vi "Write Command.vi"(8 "error in":errorcluster, 10 "command":string, 11 "GOLPI ref. in":T1={"pipe handle"={"lv_proc.dll file path"=path "", "process instance handle"=[], "debug mode"=FALSE, "debug data"=[]}, "fast read timeout [ms]"=500, "fast read settle time [ms]"=10, "fast read to multiple [ms]"=1, "max elements per input line"=100, "slow read timeout [ms]"=5000, "stdin double format specifier"="", "max elements per stdout output column"=100, "console mode bitstream"=FALSE, "bitstream first read timeout [ms]"=1000, "bitstream read timeout [ms]"=50, "struct transfer possible"=FALSE, "matlab mode"=FALSE}) -> (0 "error out":errorcluster, 3 "GOLPI ref. out":T1={"pipe handle"={"lv_proc.dll file path"=path "", "process instance handle"=[], "debug mode"=FALSE, "debug data"=[]}, "fast read timeout [ms]"=500, "fast read settle time [ms]"=10, "fast read to multiple [ms]"=1, "max elements per input line"=100, "slow read timeout [ms]"=5000, "stdin double format specifier"="", "max elements per stdout output column"=100, "console mode bitstream"=FALSE, "bitstream first read timeout [ms]"=1000, "bitstream read timeout [ms]"=50, "struct transfer possible"=FALSE, "matlab mode"=FALSE})   [LabVIEW 2020, in "GOLPI library.lvlib"]
doc: "Sends command to GNU Octave. End of line is added automatically if missing.\n\n---\nGOLPI works only with lv_proc.dll library, which is part of vipm package or should be delivered together with packed library. Placement of this dll is selected in terminal of Start GNU Octave.vi."
uses:
  GOLPI library.lvlib
  GOLPI reference Type Def.ctl
  Pipe Handle.ctl
  LV Process library.lvlib
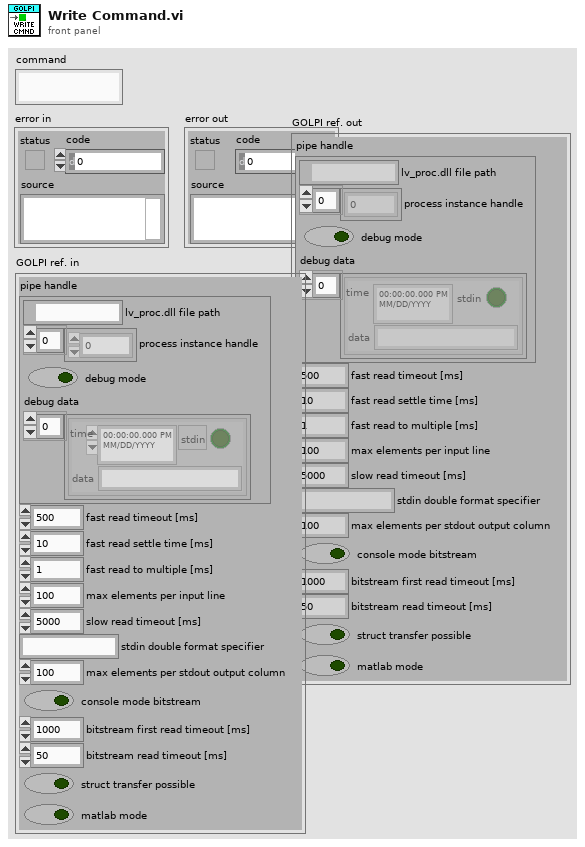
[diagram p1: front panel]
types:
  T1 = typedef "GOLPI library.lvlib/GOLPI reference Type Def.ctl" = cluster{"pipe handle":T2, "fast read timeout [ms]":u32, "fast read settle time [ms]":u32, "fast read to multiple [ms]":u32, "max elements per input line":u32, "slow read timeout [ms]":u32, "stdin double format specifier":string, "max elements per stdout output column":u32, "console mode bitstream":bool, "bitstream first read timeout [ms]":u32, "bitstream read timeout [ms]":u32, "struct transfer possible":bool, "matlab mode":bool}
  T2 = typedef "LV Process library.lvlib/Pipe Handle.ctl" = cluster{"lv_proc.dll file path":path, "process instance handle":u32[], "debug mode":bool, "debug data":cluster{"time":timestamp, "stdin":bool, "data":string}[]}
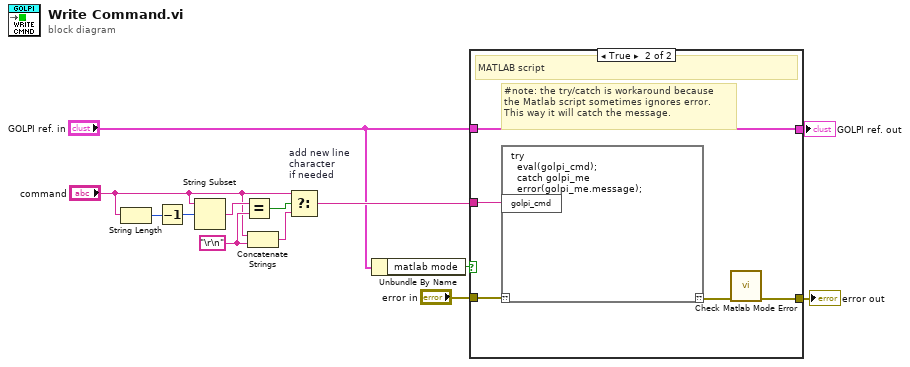
[diagram p0: block diagram]
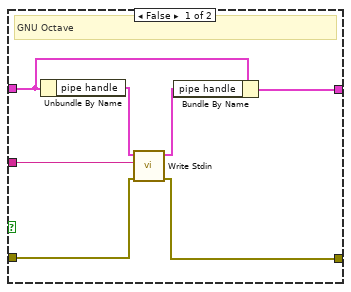
[diagram p2: hidden frame]
diagram:
  w8 = "\r\n"
  n1 = String Length(string="command") -> (length=w12:i32)
  n2 = Decrement(x=w12) -> (x-1=w11:i32)
  n3 = String Subset(string="command", offset (0)=w11) -> (substring=w10:string)  [unwired: 1 in]
  n4 = Equal?(x=w10, y=w8) -> (x = y?=w9:bool)
  n5 = Concatenate Strings("command", w8) -> (w7:string)
  n6 = Select "add new line\ncharacter\nif needed"(t="command", s=w9, f=w7) -> (s? t:f=w5:string)
  n7 = Unbundle By Name("GOLPI ref. in") -> ("matlab mode"=w1:bool)
  n8 = case shown="True" w1 {
    tunnel: "error in" -> [w20 w23]
    tunnel: w5 -> [w19 w25]
    tunnel: [w18 w21] -> w4
    tunnel: "GOLPI ref. in" -> [w17 w24]
    tunnel: [w16 w24] -> w3
    frame False {
      # "GNU Octave"
      n9 = Unbundle By Name(w17) -> ("pipe handle"=w15:T2)
      n10 = call "Write Stdin.vi"("error in"=w20, "write buffer"=w19, "pipe in"=w15) -> ("error out"=w18:errorcluster, "pipe out"=w14:T2)  [unwired: 6 in, 1 out]
      n11 = Bundle By Name(cluster=w17, "pipe handle"=w14) -> (w16:T1)
    }
    frame True {
      # "#note: the try/catch is workaround because\nthe Matlab script sometimes ignores error.\nThis way it will catch the message."
      # "MATLAB script"
      n12 = script code="try\n  eval(golpi_cmd);\n  catch golpi_me\n  error(golpi_me.message);\nend"("??"=w23, "golpi_cmd"=w25) -> ("??"=w22:errorcluster)
      n13 = call "Check Matlab Mode Error.vi"("error in"=w22) -> ("error out"=w21:errorcluster)  [unwired: 10 in]
    }
  }
  "error out" <- w4
  "GOLPI ref. out" <- w3
